vi "arange.vi"(10 "Stop":i32, 11 "Start":i32) -> (3 "Array":i32[](array[numeric]))   [LabVIEW 2019]
doc: "Creates an array from start up to but not including stop. Integers only!"
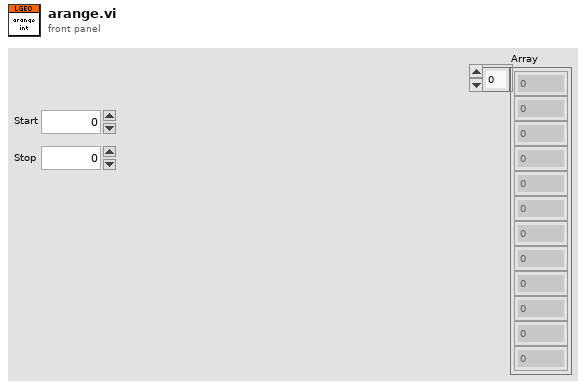
[diagram p1: front panel]
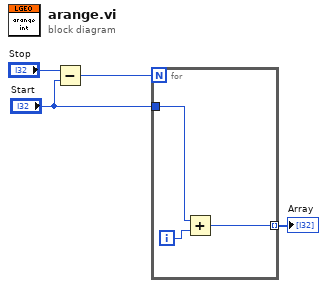
[diagram p0: block diagram]
diagram:
  n1 = Subtract(x="Stop", y="Start") -> (x-y=w4:i32)
  n2 = for {
    N: w4 -> [_]
    tunnel: [w6] -> w3 mode=indexing
    tunnel: "Start" -> [w5]
    i -> [w7]
    n3 = Add(x=w5, y=w7) -> (x+y=w6:i32)
  }
  "Array" <- w3
